vi "Parse Signal List.vi"(8 "error in":errorcluster, 11 "DAQ970 in":refnum<class "DAQ970.lvclass">) -> (0 "error out":errorcluster, 3 "DAQ970 out":refnum<class "DAQ970.lvclass">)   [LabVIEW 2019, in "DAQ970.lvlib" / "DAQ970.lvclass"]
uses:
  Library/DAQ970.lvclass
  C:/Users/Public/Documents/Development/builds/Tools/Config.lvlibp/Config.lvclass
  Library/DAQ970.lvclass/DAQ970.ctl
  builds/Tools/Config.lvlibp/Accessors/Read Device Signals.vi
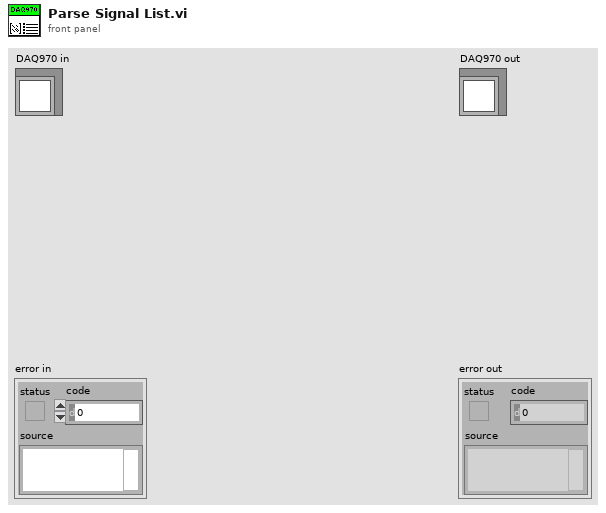
[diagram p1: front panel]
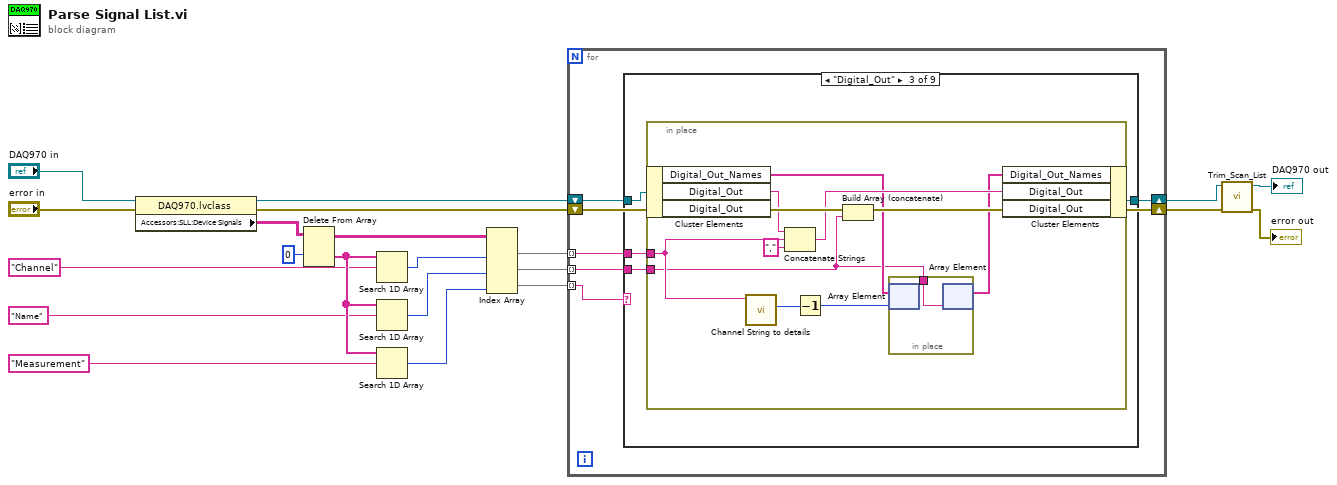
[diagram p0: block diagram]
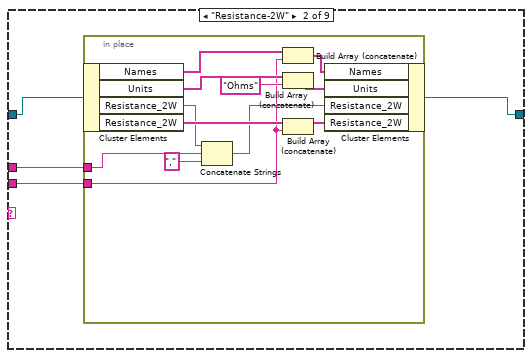
[diagram p3: hidden frame]
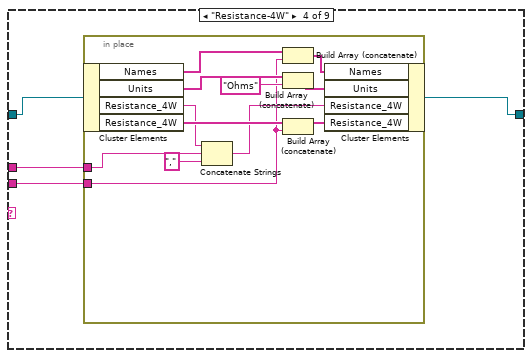
[diagram p4: hidden frame]
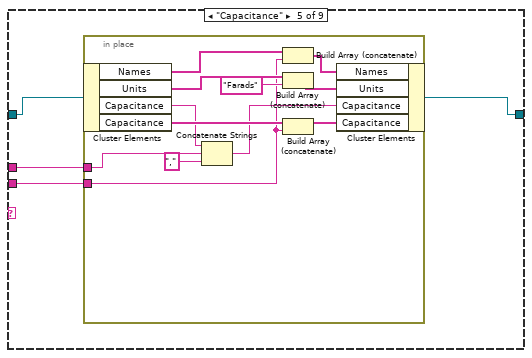
[diagram p5: hidden frame]
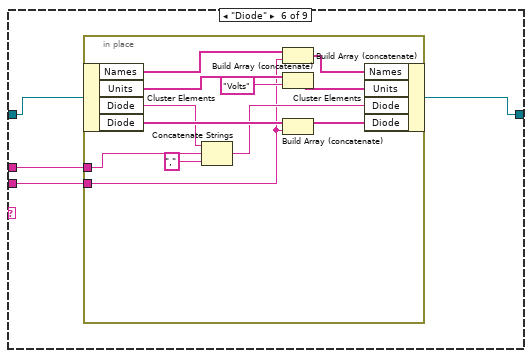
[diagram p6: hidden frame]
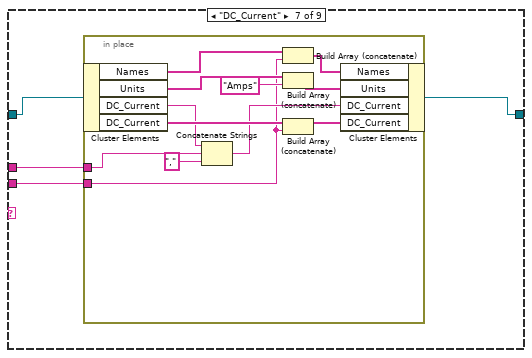
[diagram p7: hidden frame]
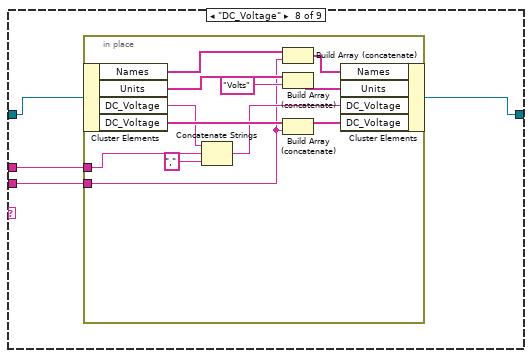
[diagram p8: hidden frame]
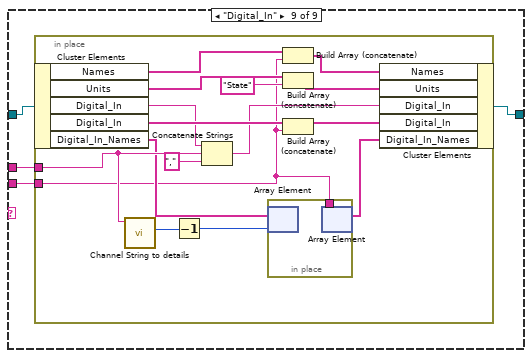
[diagram p9: hidden frame]
diagram:
  n1 = property class="DAQ970.lvclass"(reference="DAQ970 in", error in="error in") -> (reference out=w6:refnum<class "DAQ970.lvclass">, error out=w7:errorcluster, "Accessors:SLL:Device Signals"=w19:string[][])
  n2 = Delete From Array(array=w19, index (row)=0) -> (deleted portion=w17:string[], array with subset deleted=w13:string[][])  [unwired: 2 in]
  n3 = Search 1D Array(1D array=w17, element="Channel") -> (index of element=w12:i32)  [unwired: 1 in]
  n4 = Search 1D Array(1D array=w17, element="Name") -> (index of element=w11:i32)  [unwired: 1 in]
  n5 = Search 1D Array(1D array=w17, element="Measurement") -> (index of element=w10:i32)  [unwired: 1 in]
  n6 = Index Array(array=w13, index (col) #1=w12, index (col) #2=w11, index (col) #3=w10) -> (element #1=w5:string[], element #2=w9:string[], element #3=w8:string[])  [unwired: 3 in]
  n7 = for {
    shift-right: [w25] -> w4
    shift-left: w6 -> [w26]
    tunnel: w5 -> [w23] mode=indexing
    tunnel: w9 -> [w24] mode=indexing
    tunnel: w8 -> [w22] mode=indexing
    shift-right: [w27] -> w3
    shift-left: w7 -> [w27]
    n8 = case shown="\"Digital_Out\"" w22 {
      tunnel: w26 -> [w28 w32 w48 w64 w80 w96 w112 w128 w144]
      tunnel: [w28 w31 w47 w63 w79 w95 w111 w127 w143] -> w25
      tunnel: w24 -> [_ w30 w46 w62 w78 w94 w110 w126 w142]
      tunnel: w23 -> [_ w29 w45 w61 w77 w93 w109 w125 w141]
      frame "False", Default {
      }
      frame "Resistance-2W" {
        n9 = in-place {
          in-place-border: w30 -> [w34]
          in-place-border: w29 -> [w41]
          n10 = in-place-cluster #1(w32) -> ("Names"=w35:string[], "Units"=w38:string[], "Resistance_2W"=w42:string, "Resistance_2W"=w44:string[])
          n11 = Concatenate Strings(w42, w41, ",") -> (w39:string)
          n12 = Build Array (concatenate)(w35, w34) -> (w33:string[])
          n13 = Build Array (concatenate)(w38, "Ohms") -> (w36:string[])
          n14 = Build Array (concatenate)(w44, w34) -> (w43:string[])
          n15 = in-place-cluster #1("Names"=w33, "Units"=w36, "Resistance_2W"=w39, "Resistance_2W"=w43) -> (w31:refnum<class "DAQ970.lvclass">)
        }
      }
      frame "Digital_Out" {
        n16 = in-place {
          in-place-border: w46 -> [w49]
          in-place-border: w45 -> [w54]
          n17 = in-place-cluster #2(w48) -> ("Digital_Out_Names"=w51:string[], "Digital_Out"=w57:string, "Digital_Out"=w59:string[])
          n18 = call "Channel String to details.vi"("String"=w54) -> ("Channel"=w53:i32)  [unwired: 9 in, 1 out]
          n19 = Concatenate Strings(w57, w54, ",") -> (w55:string)
          n20 = Decrement(x=w53) -> (x-1=w52:i32)
          n21 = Build Array (concatenate)(w59, w49) -> (w58:string[])
          n22 = in-place {
            in-place-border: w49 -> [w60]
            n23 = in-place-array #3(w51, w52) -> ()  [unwired: 1 out]
            n24 = in-place-array #3(w60) -> (w50:string[])  [unwired: 1 out]
          }
          n25 = in-place-cluster #2("Digital_Out_Names"=w50, "Digital_Out"=w55, "Digital_Out"=w58) -> (w47:refnum<class "DAQ970.lvclass">)
        }
      }
      frame "Resistance-4W" {
        n26 = in-place {
          in-place-border: w62 -> [w66]
          in-place-border: w61 -> [w73]
          n27 = in-place-cluster #4(w64) -> ("Names"=w67:string[], "Units"=w70:string[], "Resistance_4W"=w74:string, "Resistance_4W"=w76:string[])
          n28 = Concatenate Strings(w74, w73, ",") -> (w71:string)
          n29 = Build Array (concatenate)(w67, w66) -> (w65:string[])
          n30 = Build Array (concatenate)(w70, "Ohms") -> (w68:string[])
          n31 = Build Array (concatenate)(w76, w66) -> (w75:string[])
          n32 = in-place-cluster #4("Names"=w65, "Units"=w68, "Resistance_4W"=w71, "Resistance_4W"=w75) -> (w63:refnum<class "DAQ970.lvclass">)
        }
      }
      frame "Capacitance" {
        n33 = in-place {
          in-place-border: w78 -> [w82]
          in-place-border: w77 -> [w89]
          n34 = in-place-cluster #5(w80) -> ("Names"=w83:string[], "Units"=w86:string[], "Capacitance"=w90:string, "Capacitance"=w92:string[])
          n35 = Concatenate Strings(w90, w89, ",") -> (w87:string)
          n36 = Build Array (concatenate)(w83, w82) -> (w81:string[])
          n37 = Build Array (concatenate)(w86, "Farads") -> (w84:string[])
          n38 = Build Array (concatenate)(w92, w82) -> (w91:string[])
          n39 = in-place-cluster #5("Names"=w81, "Units"=w84, "Capacitance"=w87, "Capacitance"=w91) -> (w79:refnum<class "DAQ970.lvclass">)
        }
      }
      frame "Diode" {
        n40 = in-place {
          in-place-border: w94 -> [w98]
          in-place-border: w93 -> [w105]
          n41 = in-place-cluster #6(w96) -> ("Names"=w99:string[], "Units"=w102:string[], "Diode"=w106:string, "Diode"=w108:string[])
          n42 = Concatenate Strings(w106, w105, ",") -> (w103:string)
          n43 = Build Array (concatenate)(w99, w98) -> (w97:string[])
          n44 = Build Array (concatenate)(w102, "Volts") -> (w100:string[])
          n45 = Build Array (concatenate)(w108, w98) -> (w107:string[])
          n46 = in-place-cluster #6("Names"=w97, "Units"=w100, "Diode"=w103, "Diode"=w107) -> (w95:refnum<class "DAQ970.lvclass">)
        }
      }
      frame "DC_Current" {
        n47 = in-place {
          in-place-border: w110 -> [w114]
          in-place-border: w109 -> [w121]
          n48 = in-place-cluster #7(w112) -> ("Names"=w115:string[], "Units"=w118:string[], "DC_Current"=w122:string, "DC_Current"=w124:string[])
          n49 = Concatenate Strings(w122, w121, ",") -> (w119:string)
          n50 = Build Array (concatenate)(w115, w114) -> (w113:string[])
          n51 = Build Array (concatenate)(w118, "Amps") -> (w116:string[])
          n52 = Build Array (concatenate)(w124, w114) -> (w123:string[])
          n53 = in-place-cluster #7("Names"=w113, "Units"=w116, "DC_Current"=w119, "DC_Current"=w123) -> (w111:refnum<class "DAQ970.lvclass">)
        }
      }
      frame "DC_Voltage" {
        n54 = in-place {
          in-place-border: w126 -> [w130]
          in-place-border: w125 -> [w137]
          n55 = in-place-cluster #8(w128) -> ("Names"=w131:string[], "Units"=w134:string[], "DC_Voltage"=w138:string, "DC_Voltage"=w140:string[])
          n56 = Concatenate Strings(w138, w137, ",") -> (w135:string)
          n57 = Build Array (concatenate)(w131, w130) -> (w129:string[])
          n58 = Build Array (concatenate)(w134, "Volts") -> (w132:string[])
          n59 = Build Array (concatenate)(w140, w130) -> (w139:string[])
          n60 = in-place-cluster #8("Names"=w129, "Units"=w132, "DC_Voltage"=w135, "DC_Voltage"=w139) -> (w127:refnum<class "DAQ970.lvclass">)
        }
      }
      frame "Digital_In" {
        n61 = in-place {
          in-place-border: w142 -> [w145]
          in-place-border: w141 -> [w149]
          n62 = in-place-cluster #9(w144) -> ("Names"=w152:string[], "Units"=w155:string[], "Digital_In"=w158:string, "Digital_In"=w160:string[], "Digital_In_Names"=w148:string[])
          n63 = call "Channel String to details.vi"("String"=w149) -> ("Channel"=w150:i32)  [unwired: 9 in, 1 out]
          n64 = Decrement(x=w150) -> (x-1=w146:i32)
          n65 = Concatenate Strings(w158, w149, ",") -> (w156:string)
          n66 = in-place {
            in-place-border: w145 -> [w161]
            n67 = in-place-array #10(w148, w146) -> ()  [unwired: 1 out]
            n68 = in-place-array #10(w161) -> (w147:string[])  [unwired: 1 out]
          }
          n69 = Build Array (concatenate)(w152, w145) -> (w151:string[])
          n70 = Build Array (concatenate)(w155, "State") -> (w153:string[])
          n71 = Build Array (concatenate)(w160, w145) -> (w159:string[])
          n72 = in-place-cluster #9("Names"=w151, "Units"=w153, "Digital_In"=w156, "Digital_In"=w159, "Digital_In_Names"=w147) -> (w143:refnum<class "DAQ970.lvclass">)
        }
      }
    }
  }
  n73 = call "Trim_Scan_List.vi"("error in"=w3, "DAQ970 in"=w4) -> ("error out"=→"error out":errorcluster, "DAQ970 out"=→"DAQ970 out":refnum<class "DAQ970.lvclass">)  [unwired: 8 in]
